vi "getRegisters.vi"(0 "AddressSpace in":refnum<class "AddressSpace.lvclass">) -> (4 "AddressSpace out":refnum<class "AddressSpace.lvclass">, 6 "LimitsRegisters":T1={"HighLimits"="HighLimits", "LowLimits"="LowLimits", "ClearLimits"="ClearLimits", "LimitsFlag"="ClearLimits"}, 8 "ConfigRegisters":T2)   [LabVIEW 2015, in "ScaleAndLimit.lvlib" / "AddressSpace.lvclass"]
uses:
  AddressSpace.lvclass
  ConfigRegisters.ctl
  LimitsRegisters.ctl
  AddressSpace.lvclass/AddressSpace.ctl
  ScaleAndLimit.lvlib
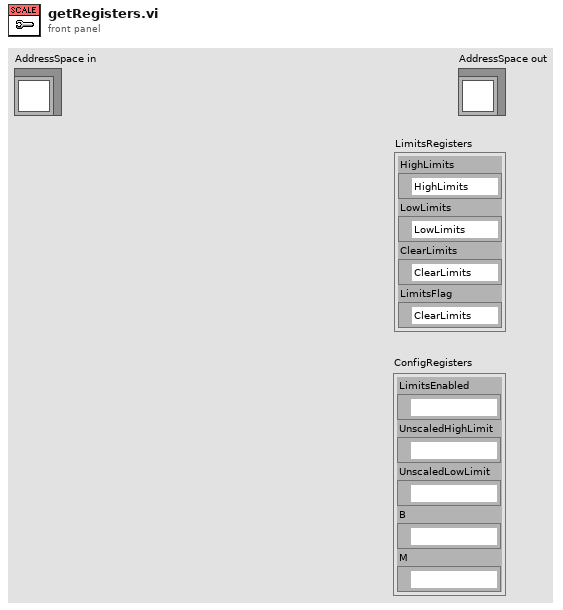
[diagram p1: front panel]
types:
  T1 = typedef "ScaleAndLimit.lvlib/LimitsRegisters.ctl" = cluster{"HighLimits":refnum<k21>, "LowLimits":refnum<k21>, "ClearLimits":refnum<k21>, "LimitsFlag":refnum<k21>}
  T2 = typedef "ScaleAndLimit.lvlib/ConfigRegisters.ctl" = cluster{"LimitsEnabled":refnum<k21>, "UnscaledHighLimit":refnum<k21>, "UnscaledLowLimit":refnum<k21>, "B":refnum<k21>, "M":refnum<k21>}
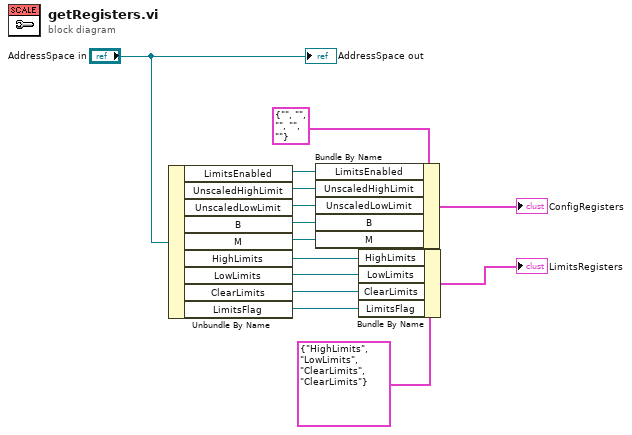
[diagram p0: block diagram]
diagram:
  n1 = Unbundle By Name("AddressSpace in") -> ("LimitsEnabled"=w9:refnum<k21>, "UnscaledHighLimit"=w10:refnum<k21>, "UnscaledLowLimit"=w11:refnum<k21>, "B"=w12:refnum<k21>, "M"=w13:refnum<k21>, "HighLimits"=w5:refnum<k21>, "LowLimits"=w4:refnum<k21>, "ClearLimits"=w2:refnum<k21>, "LimitsFlag"=w1:refnum<k21>)
  n2 = Bundle By Name(cluster=T2 {"LimitsEnabled"="", "UnscaledHighLimit"="", "UnscaledLowLimit"="", "B"="", "M"=""} ("ConfigRegisters"), "LimitsEnabled"=w9, "UnscaledHighLimit"=w10, "UnscaledLowLimit"=w11, "B"=w12, "M"=w13) -> (→"ConfigRegisters":T2)
  n3 = Bundle By Name(cluster=T1 {"HighLimits"="HighLimits", "LowLimits"="LowLimits", "ClearLimits"="ClearLimits", "LimitsFlag"="ClearLimits"} ("LimitsRegisters"), "HighLimits"=w5, "LowLimits"=w4, "ClearLimits"=w2, "LimitsFlag"=w1) -> (→"LimitsRegisters":T1)
  "AddressSpace out" <- "AddressSpace in"
